vi "Run.vi"(8 "error in (no error)":errorcluster caption="entrée d'erreur (pas d'erreur)", 9 "Y":string[][](array[string]), 10 "X":string[][](array[string]), 11 "Nan_euclidean_distances.lvclass":refnum<class "Nan_euclidean_distances.lvclass">) -> (0 "error out":errorcluster caption="sortie d'erreur", 2 "Data":T1, 3 "Nan_euclidean_distances.lvclass":refnum<class "Nan_euclidean_distances.lvclass">)   [LabVIEW 2020, in "Nan_euclidean_distances.lvclass"]
doc: "Returns : \n\n- distances : array, shape (n_samples_1, n_samples_2)"
uses:
  Nan_euclidean_distances.lvclass
  Nan_euclidean_distances.lvclass/Nan_euclidean_distances.ctl
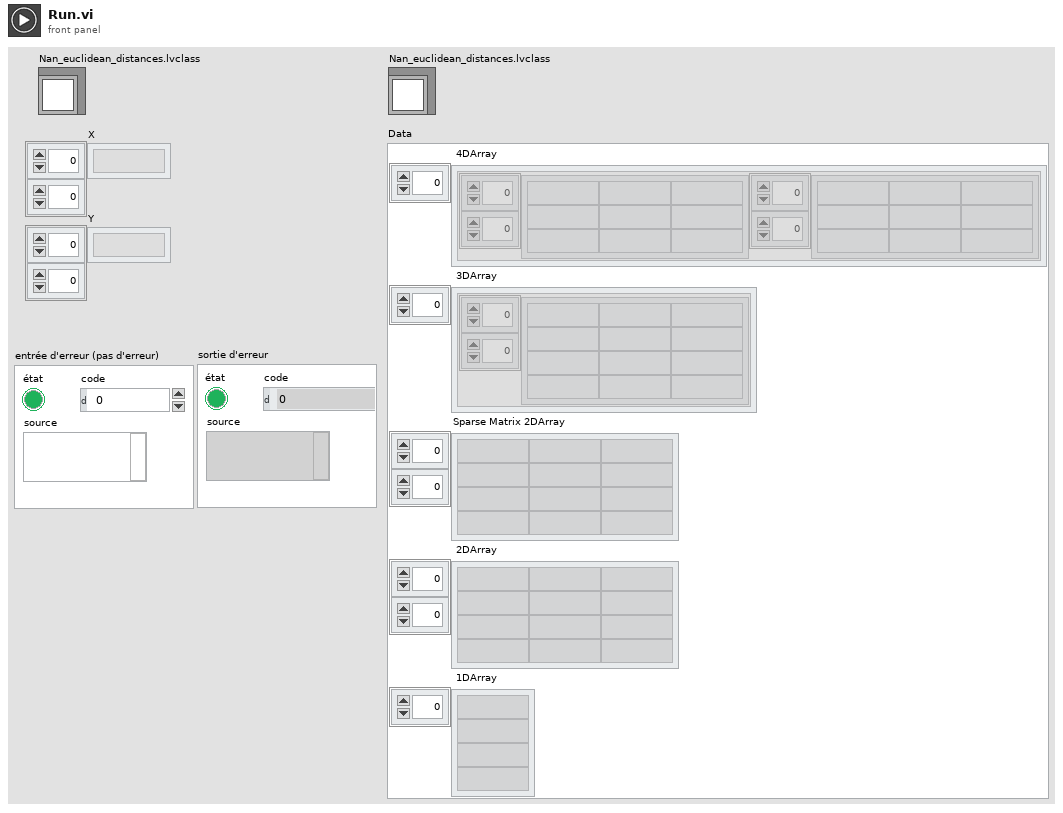
[diagram p1: front panel]
types:
  T1 = cluster{" 4DArray":cluster{"1":string[][], "2":string[][]}[], " 3DArray":cluster{"Tableau":string[][]}[], "Sparse Matrix 2DArray":string[][], " 2DArray":string[][], " 1DArray":string[]}
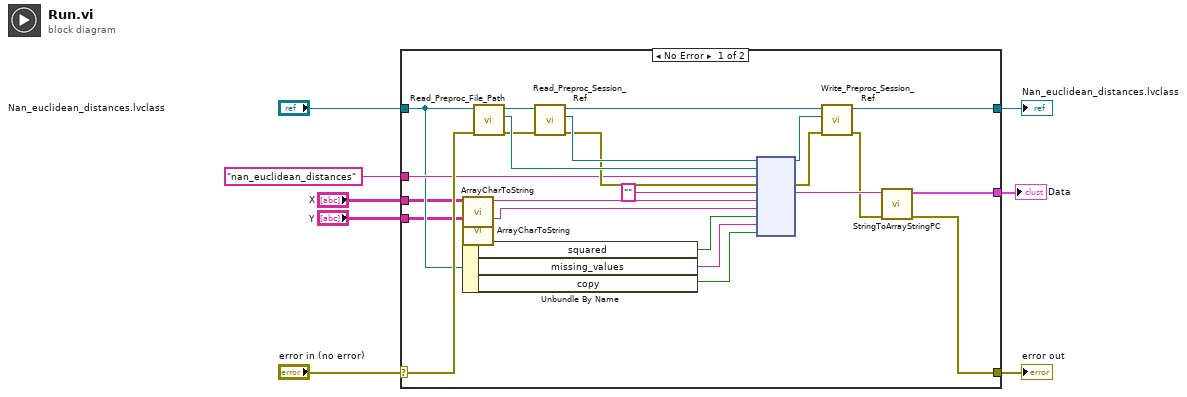
[diagram p0: block diagram]
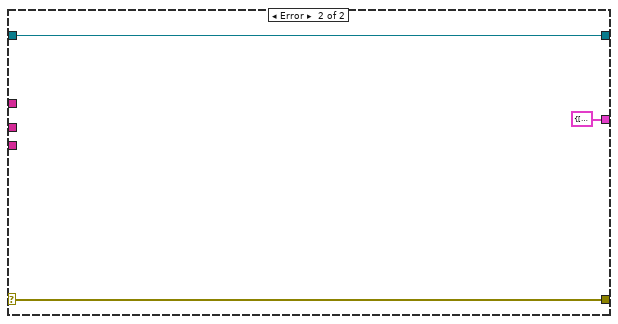
[diagram p2: hidden frame]
diagram:
  n1 = case shown="No Error" "error in (no error)" {
    selector: "error in (no error)" -> [w23 w35]
    tunnel: [w10 w35] -> w7
    tunnel: [w13 w34] -> w5
    tunnel: "Nan_euclidean_distances.lvclass" -> [w21 w34]
    tunnel: "nan_euclidean_distances" ("Fonction") -> [w22 _]
    tunnel: "X" -> [w17 _]
    tunnel: "Y" -> [w16 _]
    tunnel: [w9 T1 {" 4DArray"=[], " 3DArray"=[], "Sparse Matrix 2DArray"=[], " 2DArray"=[], " 1DArray"=[]} ("Data")] -> w1
    frame No Error {
      n2 = call "ArrayCharToString.vi"("TAB"=w17) -> ("Instruction"=w15:string)  [unwired: 10 in]
      n3 = call "ArrayCharToString.vi"("TAB"=w16) -> ("Instruction"=w14:string)  [unwired: 10 in]
      n4 = Unbundle By Name(w21) -> ("squared"=w20:bool, "missing_values"=w19:string, "copy"=w18:bool)
      n5 = call-dynamic "Read_Preproc_File_Path.vi"("error in (no error)"=w23, "Python in"=w21) -> ("error out"=w27:errorcluster, "File_Path"=w30:path, "Python out"=w32:refnum<class "Nan_euclidean_distances.lvclass">)  [unwired: 7 in]
      n6 = call-dynamic "Read_Preproc_Session_Ref.vi"("error in (no error)"=w27, "Python in"=w32) -> ("error out"=w28:errorcluster, "Session_ref"=w29:refnum<k35>, "Python out"=w31:refnum<class "Nan_euclidean_distances.lvclass">)  [unwired: 7 in]
      n7 = node(w29, w30, w22, w28, "", w15, w14, w20, w19, w18) -> (w24:refnum<k35>, w26:errorcluster, w12:string)  [unwired: 5 in, 2 out]
      n8 = call-dynamic "Write_Preproc_Session_Ref.vi"("error in (no error)"=w26, "Session_ref"=w24, "Python in"=w31) -> ("error out"=w11:errorcluster, "Python out"=w13:refnum<class "Nan_euclidean_distances.lvclass">)  [unwired: 7 in]
      n9 = call "StringToArrayStringPC.vi"("sortie d'erreur"=w11, "Return value"=w12) -> ("sortie d'erreur"=w10:errorcluster, "Data"=w9:T1)  [unwired: 8 in]
    }
    frame Error {
    }
  }
  "error out" <- w7
  "Nan_euclidean_distances.lvclass" <- w5
  "Data" <- w1
